vi "Read IConfigure.vi"(8 "error in (no error)":errorcluster, 11 "Scope Base in":refnum<class "Scope Base.lvclass">) -> (0 "error out":errorcluster, 2 "IConfigureScope":refnum<class "IConfigure.lvclass">, 3 "Scope Base out":refnum<class "Scope Base.lvclass">)   [LabVIEW 2023, in "Scope.lvlib" / "Scope Base.lvlib" / "Scope Base.lvclass"]
uses:
  Scope Base.lvclass
  Interfaces/IConfigure/IConfigure.lvclass
  Scope Base.lvclass/Scope Base.ctl
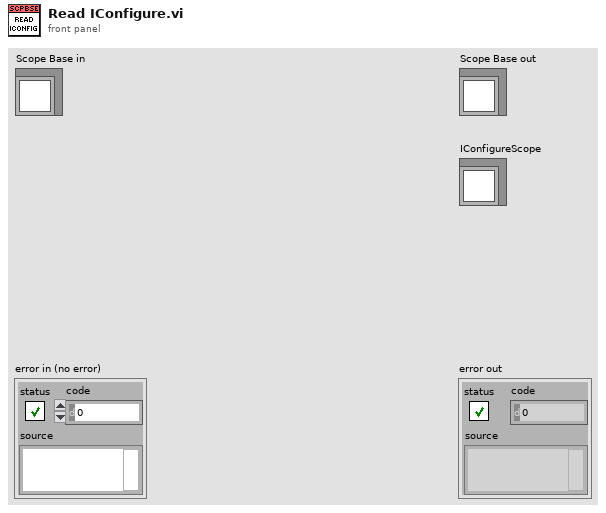
[diagram p1: front panel]
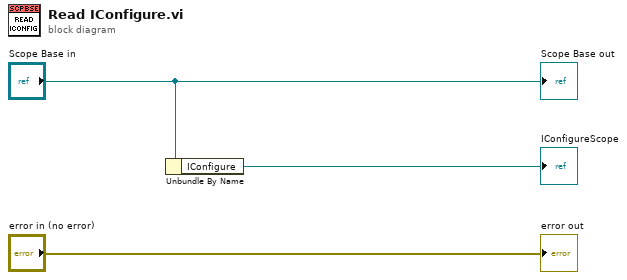
[diagram p0: block diagram]
diagram:
  n1 = Unbundle By Name("Scope Base in") -> ("IConfigure"=→"IConfigureScope":refnum<class "IConfigure.lvclass">)
  "error out" <- "error in (no error)"
  "Scope Base out" <- "Scope Base in"
